vi "Tell Parent.vi"(4 "Priority":bool, 7 "Actor in":refnum<class "Actor.lvclass">) -> (0 "Error out":errorcluster)   [LabVIEW 2025, in "_Template.lvlib" / "Templates.lvlib" / "TEMPLATE Msg.lvlib"]
uses:
  TEMPLATE Msg.lvlib
  jettl/jettl/Actor/Actor.lvclass
  TEMPLATE Msg/TEMPLATE Msg.lvclass
  jettl/jettl/jettl.lvlib
panel:
  # "This front panel should not be manipulated."
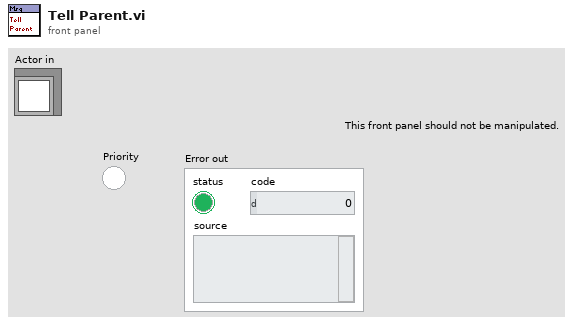
[diagram p1: front panel]
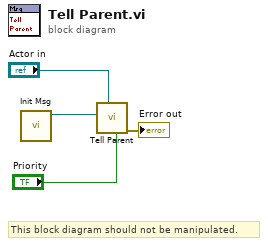
[diagram p0: block diagram]
diagram:
  # "This block diagram should not be manipulated."
  n1 = call "Init Msg.vi"() -> ("TEMPLATE Msg out"=w2:refnum<class "TEMPLATE Msg.lvclass">)  [unwired: 11 in]
  n2 = call "Tell Parent.vi"("Priority"="Priority", "Actor in"="Actor in", "Msg"=w2) -> ("Error out"=→"Error out":errorcluster)  [unwired: 8 in]
